vi "Validate Configuration.vi"(8 "error in":errorcluster, 11 "IValidateConfiguration in":refnum<class "IMAQdx Base Configure Strategy.lvclass">) -> (0 "error out":errorcluster, 3 "IValidateConfiguration out":refnum<class "IMAQdx Base Configure Strategy.lvclass">)   [LabVIEW 2024, in "IMAQdx Base Configure Strategy.lvclass"]
uses:
  IMAQdx Base Configure Strategy.lvclass
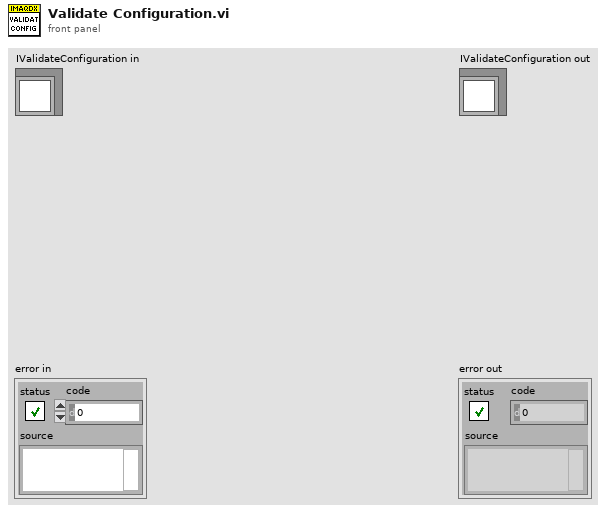
[diagram p1: front panel]
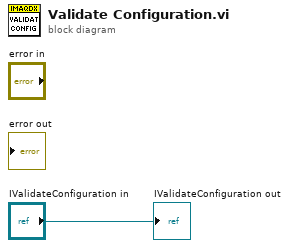
[diagram p0: block diagram]
diagram:
  "IValidateConfiguration out" <- "IValidateConfiguration in"
